vi "CLIENT-KILL.vi"(0 "refnum in":refnum<vi>, 5 "IP":string, 7 "Port":string, 11 "error in":errorcluster) -> (4 "refnum out":refnum<vi>, 6 "Data":T1, 15 "error out":errorcluster)   [LabVIEW 2023]
uses:
  SubVIs/Controls/redis-data.ctl
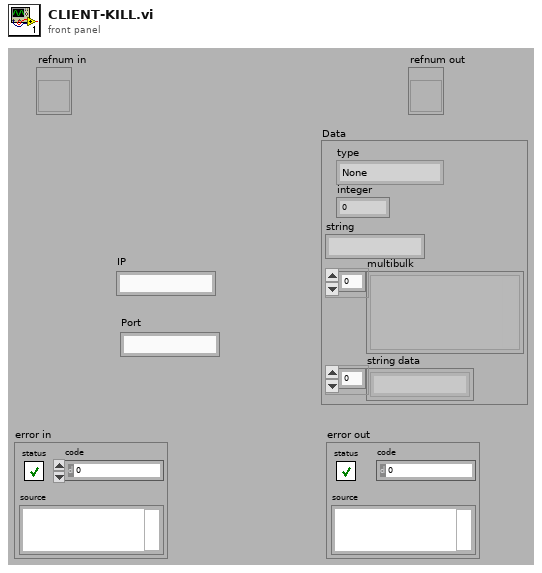
[diagram p1: front panel]
types:
  T1 = typedef "redis-data.ctl" = cluster{"type":enum16{"None", "Error", "Status", "Nil", "Integer", "String", "Multibulk"}, "integer":i64, "string":string, "multibulk":variant[], "string data":string[]}
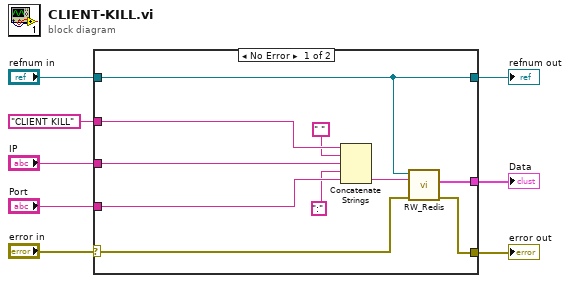
[diagram p0: block diagram]
diagram:
  n1 = case shown="No Error" "error in" {
    selector: "error in" -> [w16 w20]
    tunnel: "IP" -> [w13 _]
    tunnel: "CLIENT KILL" -> [w18 _]
    tunnel: "refnum in" -> [w10 w19]
    tunnel: [w15 w20] -> w6
    tunnel: [w14 _] -> w1
    tunnel: "Port" -> [w11 _]
    tunnel: [w10 w19] -> w2
    frame No Error {
      n2 = Concatenate Strings(w18, " ", w13, ":", w11) -> (w17:string)
      n3 = call "RW_Redis.vi"("error in"=w16, "command"=w17, "TCP session in"=w10) -> ("error out"=w15:errorcluster, "Data"=w14:T1)  [unwired: 6 in, 1 out]
    }
    frame Error {
    }
  }
  "error out" <- w6
  "refnum out" <- w2
  "Data" <- w1
